vi "MListbox Autosize Column Width.vi"(8 "error in (no error)":errorcluster, 11 "Multicolumn ListBox in":refnum<class "Multicolumn ListBox.lvclass">) -> (0 "error out":errorcluster, 3 "Multicolumn ListBox out":refnum<class "Multicolumn ListBox.lvclass">)   [LabVIEW 2018]
uses:
  Multicolumn ListBox.lvclass
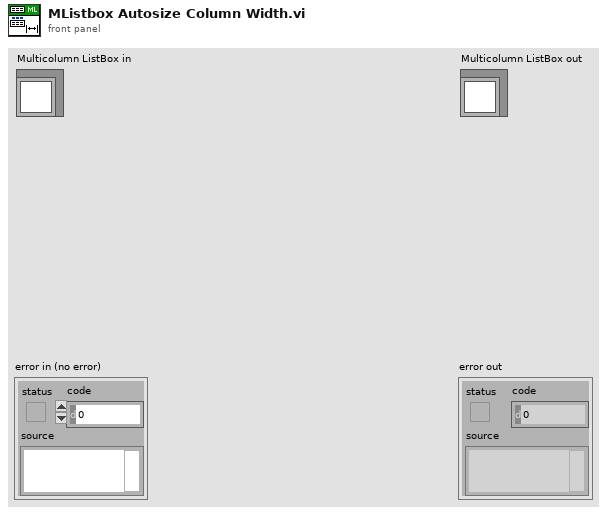
[diagram p1: front panel]
types:
  T1 = cluster{"left":i16, "top":i16, "right":i16, "bottom":i16}
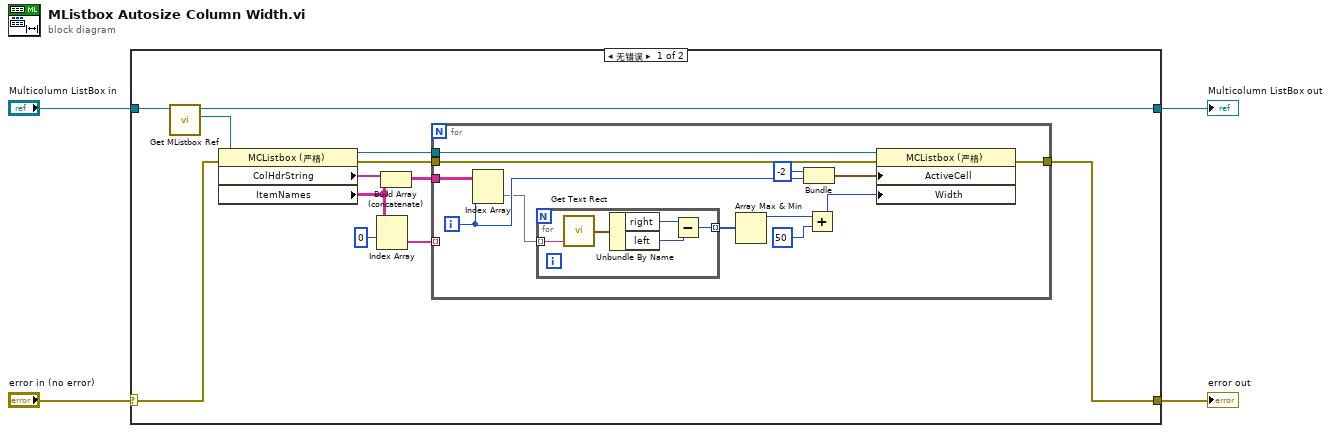
[diagram p0: block diagram]
diagram:
  n1 = case shown="无错误" "error in (no error)" {
    selector: "error in (no error)" -> [w13 w35]
    tunnel: [w10 w35] -> w3
    tunnel: [w15 w34] -> w1
    tunnel: "Multicolumn ListBox in" -> [w16 w34]
    frame No Error {
      n2 = call "Get MListbox Ref.vi"("Multicolumn ListBox in"=w16) -> ("MListbox Ref"=w14:refnum<vi>, "Multicolumn ListBox out"=w15:refnum<class "Multicolumn ListBox.lvclass">)  [unwired: 8 in, 1 out]
      n3 = property class="MCListbox (严格)"(reference=w14, error in=w13) -> (reference out=w12:refnum<vi>, error out=w11:errorcluster, "ColHdrString"=w7:string[], "ItemNames"=w6:string[][])
      n4 = Index Array(array=w6, index (row)=0 ("索引 (行)")) -> (element=w8:string[])  [unwired: 1 in]
      n5 = Build Array (concatenate)(w7, w6) -> (w5:string[][])
      n6 = for {
        tunnel: w12 -> [w28]
        tunnel: w11 -> [w27]
        tunnel: [w22] -> w10
        tunnel: w8 -> [_] mode=indexing
        tunnel: w5 -> [w21]
        i -> [w20]
        n7 = Index Array(array=w21, index (col)=w20) -> (element=w19:string[])  [unwired: 1 in]
        n8 = for {
          tunnel: [w30] -> w18 mode=indexing
          tunnel: w19 -> [w29] mode=indexing
          n9 = call <vilib>:"Get Text Rect.vi"("text"=w29) -> ("rect"=w33:T1)  [unwired: 8 in]
          n10 = Unbundle By Name(w33) -> ("right"=w32:i16, "left"=w31:i16)
          n11 = Subtract(x=w32, y=w31) -> (x-y=w30:i16)
        }
        n12 = Array Max & Min(array=w18) -> (max value=w17:i16)  [unwired: 3 out]
        n13 = Bundle("Row"=-2, w20) -> (w23:cluster{"Row":i32, i32})  [unwired: 1 in]
        n14 = Add(x=w17, y=50) -> (x+y=w25:i32)
        n15 = property class="MCListbox (严格)"(reference=w28, error in=w27, "ActiveCell"=w23, "Width"=w25) -> (error out=w22:errorcluster)  [unwired: 1 out]
      }
    }
    frame Error {
    }
  }
  "error out" <- w3
  "Multicolumn ListBox out" <- w1
